vi "Configuration Tool Main.vi"() -> ()   [LabVIEW 2013, in "Configuration Tool.lvlib"]
doc: "This is the main VI for the configuration editor."
uses:
  Configuration Tool.lvlib
  Controls/StateCluster.ctl
  Configuration Framework/Repository/NISE_CEF_Repository.lvclass
  Configuration Framework/Node/NodeRef.ctl
  Configuration Framework/Node/NISE_CEF_Node.lvclass
  Configuration Framework/Node/StandardEvents.ctl
  Configuration Framework/Node/UserEventRef.ctl
  Configuration Framework/Controls/EventCluster.ctl
  Configuration Framework/Node/NodeChangeEvent.ctl
  Configuration Framework/Node/CacheState.ctl
  Configuration Framework/Node/RefreshUIEvent.ctl
  Configuration Framework/Node/StopEvent.ctl
  Configuration Framework/glyph manager/glyph manager.ctl
  <vilib>/picture/picture.llb/imagedata.ctl
  Controls/AddMessage.ctl
  Controls/MoveMessage.ctl
  <vilib>/Utility/error.llb/DialogType.ctl
  Classes/cRIO/cRIO.lvclass
  Classes/cRIO Repo/cRIORepo.lvclass
  <vilib>/Utility/sysdir.llb/System Directory Type.ctl
  <vilib>/NI/AMC/Read Termination Message.vi
  <vilib>/NI/AMC/Create Single Message.vi
  <vilib>/NI/AMC/Update Message Routing Info.vi
  <vilib>/NI/AMC/Send Message.vi
  <vilib>/NI/AMC/Globals.vi
  <vilib>/NI/AMC/AMC.lvlib
  Configuration Framework/NISE_CEF_TreeControl.lvlib
  Configuration Framework/glyph manager/glyph manager.lvlib
panel:
  in  "View":string(tree)
  in  "Exit":bool
  # "Configurator"
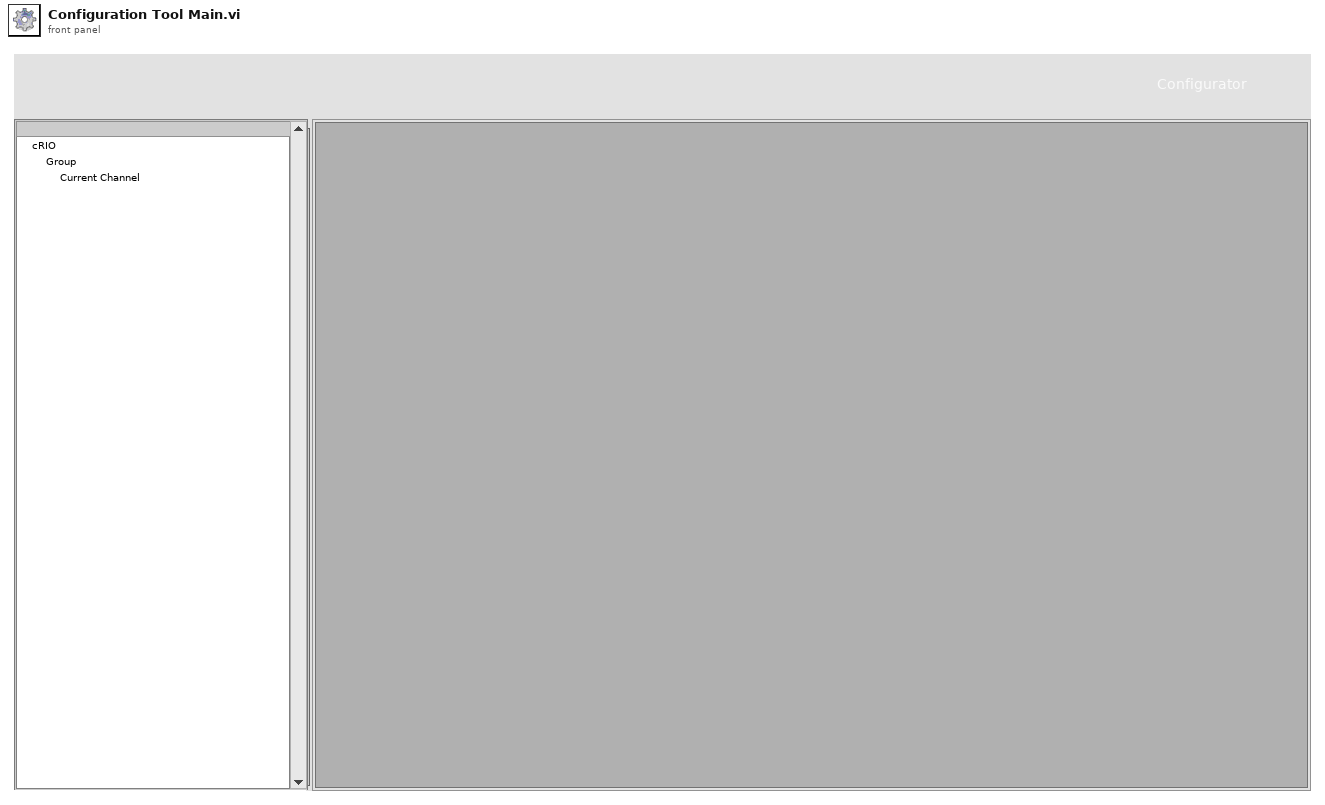
[diagram p1: front panel]
types:
  T1 = typedef "Configuration Tool.lvlib/StateCluster.ctl" = cluster{"repository":refnum<class "NISE_CEF_Repository.lvclass">, "root":T2, "unsaved changes":bool, "current path":path, "standard events":T3, "classes path":path, "glyph manager":T9}
  T2 = typedef "NISE_CEF_Node.lvclass/NodeRef.ctl" = refnum<data-value>
  T3 = typedef "NISE_CEF_Node.lvclass/StandardEvents.ctl" = cluster{"user event":T4, "node change":T5, "cache state":T6, "refresh UI":T7, "stop event":T8}
  T4 = typedef "NISE_CEF_Node.lvclass/UserEventRef.ctl" = refnum<user-event>
  T5 = typedef "NISE_CEF_Node.lvclass/NodeChangeEvent.ctl" = refnum<user-event>
  T6 = typedef "NISE_CEF_Node.lvclass/CacheState.ctl" = refnum<user-event>
  T7 = typedef "NISE_CEF_Node.lvclass/RefreshUIEvent.ctl" = refnum<user-event>
  T8 = typedef "NISE_CEF_Node.lvclass/StopEvent.ctl" = refnum<user-event>
  T9 = typedef "glyph manager.lvlib/glyph manager.ctl" = cluster{"search paths":path[], "glyph map":variant, "base glyphs":T10[], "desired overlays":string[]}
  T10 = typedef "imagedata.ctl" = cluster{"image type":i32, "image depth":i32, "image":u8[], "mask":u8[], "colors":u32[], "Rectangle":cluster{"left":i16, "top":i16, "right":i16, "bottom":i16}}
  T11 = typedef "AMC.lvlib/Message Queue.ctl" = refnum<queue>
  T12 = typedef "Configuration Tool.lvlib/AddMessage.ctl" = cluster{"node type":string, "to add to":string}
  T13 = typedef "Configuration Tool.lvlib/MoveMessage.ctl" = cluster{"node ref":T2, "new parent":T2}
  T14 = typedef "Configuration Tool.lvlib/FilePaths.ctl" = cluster{"glyphs":path, "classes":path}
  T15 = typedef "DialogType.ctl" = u16
  T16 = typedef "System Directory Type.ctl" = i32
  T17 = typedef "NISE_CEF_Node.lvclass/Summary.ctl" = cluster{"ID":string, "parent ID":string, "node type":string, "text":string, "additional text":string, "glyph":string, "depth":i32, "glyph overlay":string}
  T18 = typedef "LVPoint32TypeDef.ctl" = cluster{"Horizontal":i32, "Vertical":i32}
  T19 = cluster{"data name":string, "drag data":variant}[]
  T20 = typedef "NISE_CEF_Node.lvclass/NodeMenuOptions.ctl" = cluster{"removable":bool, "movable":bool, "duplicate":bool}
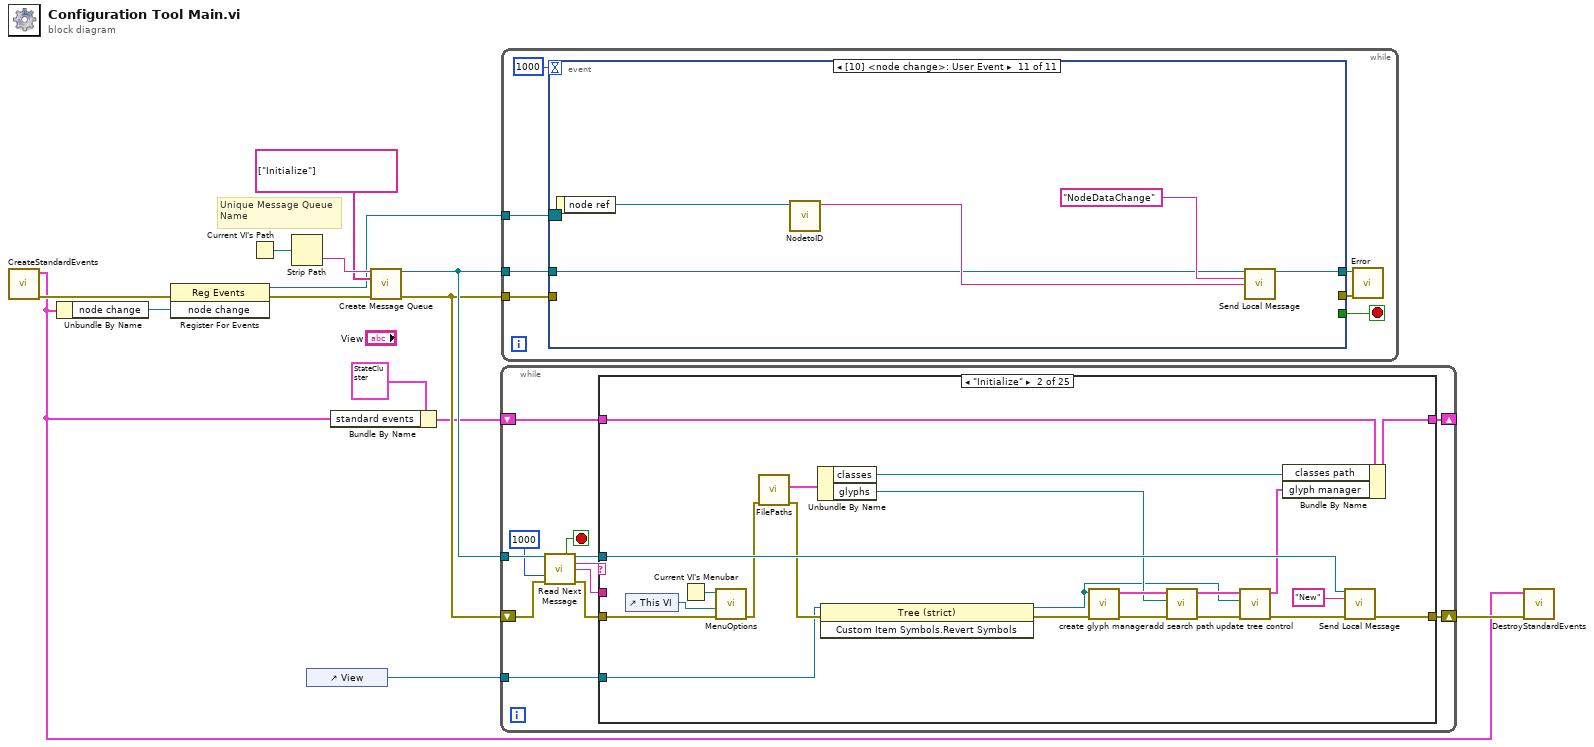
[diagram p0: block diagram]
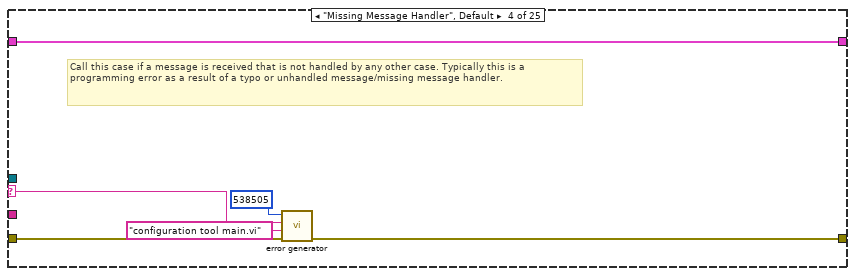
[diagram p4: hidden frame]
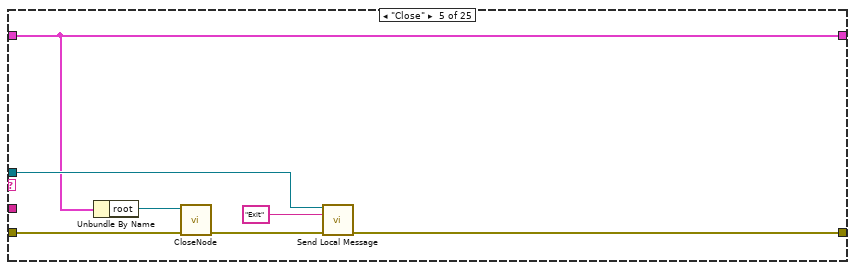
[diagram p5: hidden frame]
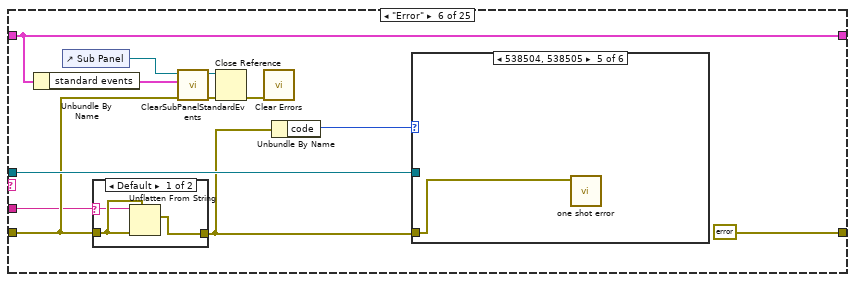
[diagram p6: hidden frame]
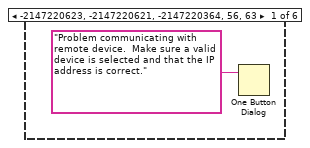
[diagram p8: hidden frame]
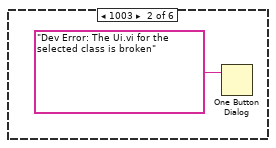
[diagram p9: hidden frame]
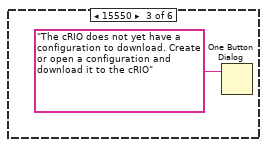
[diagram p10: hidden frame]
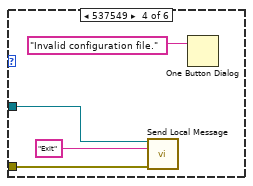
[diagram p11: hidden frame]
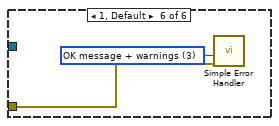
[diagram p12: hidden frame]
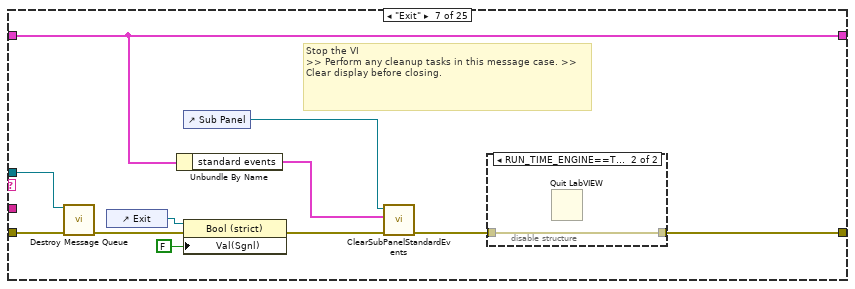
[diagram p13: hidden frame]
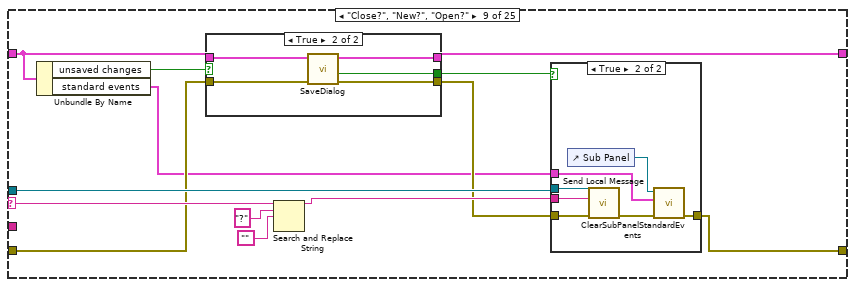
[diagram p16: hidden frame]
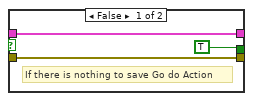
[diagram p17: hidden frame]
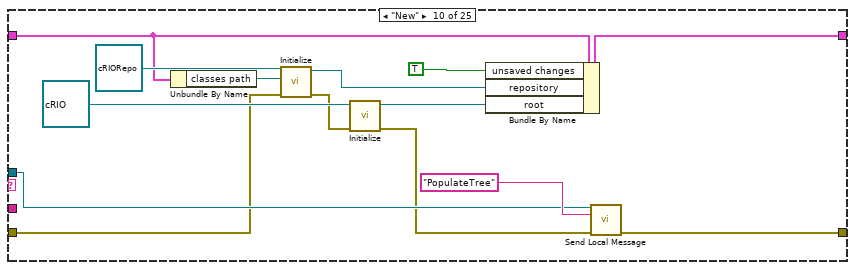
[diagram p19: hidden frame]
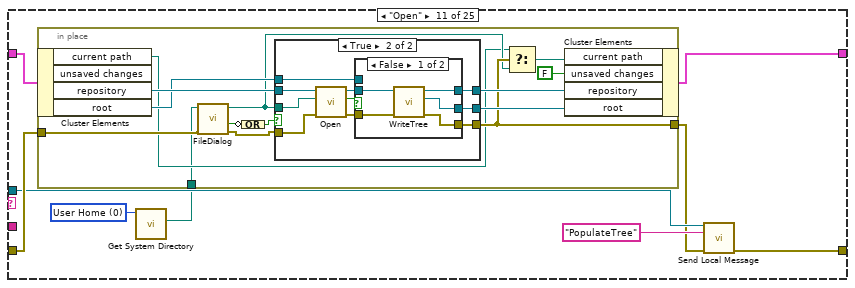
[diagram p20: hidden frame]
diagram:
  # "Unique Message Queue Name"
  n1 = call "CreateStandardEvents.vi"() -> ("error out"=w9:errorcluster, "standard events"=w3:T3)  [unwired: 10 in]
  n2 = Unbundle By Name(w3) -> ("node change"=w8:T5)
  n3 = register-events(error in=w9, w8) -> (reference out=w2:refnum<event-registration>, error out=w7:errorcluster)  [unwired: 1 in]
  n4 = Current VI's Path() -> (path=w13:path)
  n5 = Strip Path(path=w13) -> (name=w14:string)  [unwired: 1 out]
  n6 = control-ref of="View"() -> (w1:refnum<vi>)
  n7 = Bundle By Name(cluster=T1 {"repository"=refnum, "root"=refnum, "unsaved changes"=FALSE, "current path"=path "", "standard events"={"user event"=refnum, "node change"=refnum, "cache state"=refnum, "refresh UI"=refnum, "stop event"=refnum}, "classes path"=path "", "glyph manager"={"search paths"=[], "glyph map"=variant, "base glyphs"=[], "desired overlays"=[]}}, "standard events"=w3) -> (w5:T1)
  n8 = call <vilib>:"Create Message Queue.vi"("message queue name"=w14, "initial message names"=string[] ["Initialize"], "error in"=w7) -> ("message queue out"=w11:T11, "error out"=w10:errorcluster)  [unwired: 11 in]
  n9 = while "Message Processor" {
    shift-right: [w22] -> w4
    shift-left: w10 -> [w21]
    tunnel: w11 -> [w20]
    shift-right: [w18] -> _
    shift-left: w5 -> [w17]
    tunnel: w1 -> [w15]
    stop <- w26 stop-if-true
    n10 = call <vilib>:"Read Next Message.vi"("message queue in"=w20, "timeout (1 ms)"=1000, "error in"=w21) -> ("exit process?"=w26:bool, "message queue out"=w16:T11, "message name"=w25:string, "message value"=w24:string, "error out"=w23:errorcluster)  [unwired: 5 in, 3 out]
    n11 = case shown="\"Initialize\"" w25 {
      selector: w25 -> [_ _ _ w54 _ _ _ _ w115 _ _ _ _ _ _ _ _ w312 _ _ _ _ _ _ _]
      tunnel: w24 -> [_ _ _ _ _ w67 _ _ _ _ _ _ _ w230 _ w273 w290 w310 w349 w373 _ _ w412 w432 w439]
      tunnel: w23 -> [w28 w50 w52 w57 w60 w70 w102 w106 w108 w136 w156 w196 w222 w237 w250 w265 w289 w315 w351 w372 w393 w402 w411 w430 w440]
      tunnel: [w28 w46 w52 w55 w64 errorcluster {"status"=FALSE, "code"=0, "source"=""} ("error out") w94 w106 w119 w148 w152 w200 w224 w234 w250 w267 w293 w318 w354 w369 w387 w398 w408 w425 w438] -> w22
      tunnel: [w27 w42 w51 w58 w62 w74 w93 w105 w110 w146 w157 w203 w223 w231 w249 w259 w286 w319 w353 w374 w383 w401 w406 w433 w435] -> w18
      tunnel: w17 -> [w27 w43 w51 w58 w62 w74 w93 w105 w111 w140 w158 w198 w221 w232 w249 w263 w287 w319 w344 w374 w396 w401 w406 w433 w441]
      tunnel: w16 -> [_ w45 _ _ w63 w77 w101 _ w118 w147 w154 w199 _ w233 _ _ _ w313 _ _ _ _ w407 w424 w437]
      tunnel: w15 -> [_ w29 _ _ _ _ _ _ _ _ _ _ _ _ _ w260 w282 w307 w346 w367 w385 _ _ _ _]
      frame "------------Generic Operations------------" {
        # "Dummy case to add a seperation in the Case Structure menu"
      }
      frame "Initialize" {
        n12 = control-ref of="This VI"() -> (w49:refnum<vi>)
        n13 = Current VI's Menubar() -> (w48:refnum<k9>)
        n14 = call "MenuOptions.vi"("error in"=w50, "VI ref"=w49, "menu ref in"=w48) -> ("error out"=w41:errorcluster)  [unwired: 7 in, 1 out]
        n15 = call "FilePaths.vi"("error in"=w41) -> ("error out"=w32:errorcluster, "paths"=w44:T14)  [unwired: 9 in]
        n16 = Unbundle By Name(w44) -> ("classes"=w40:path, "glyphs"=w34:path)
        n17 = invoke class="Tree (strict)" method="Custom Item Symbols.Revert Symbols"(reference=w29, error in=w32) -> (reference out=w30:refnum<vi>, error out=w31:errorcluster)  [unwired: 1 in, 1 out]
        n18 = call "create glyph manager.vi"("error in"=w31, "tree ref (for default symbols)"=w30) -> ("error out"=w39:errorcluster, "glyph manager"=w38:T9)  [unwired: 8 in]
        n19 = call "add search path.vi"("error in"=w39, "search path"=w34, "glyph manager in"=w38) -> ("error out"=w37:errorcluster, "glyph manager out"=w36:T9)  [unwired: 7 in]
        n20 = call "update tree control.vi"("error in"=w37, "tree reference"=w30, "glyph manager in"=w36) -> ("error out"=w35:errorcluster, "glyph manager out"=w33:T9)  [unwired: 7 in]
        n21 = Bundle By Name(cluster=w43, "classes path"=w40, "glyph manager"=w33) -> (w42:T1)
        n22 = call <vilib>:"Send Local Message.vi"("message queue in"=w45, "message name"="New" ("Message Name"), "error in"=w35) -> ("error out"=w46:errorcluster)  [unwired: 10 in, 2 out]
      }
      frame "", "Idle" {
      }
      frame "Missing Message Handler", Default {
        # "Call this case if a message is received that is not handled by any other case. Typically this is a programming error as a result of a typo or unhandled message/missing message handler."
        n23 = call "error generator.vi"("error in"=w57, "source"="configuration tool main.vi", "append error message"=w54, "error code (0)"=538505) -> ("error out"=w55:errorcluster)  [unwired: 5 in]
      }
      frame "Close" {
        n24 = Unbundle By Name(w62) -> ("root"=w61:T2)
        n25 = call "CloseNode.vi"("error in"=w60, "node ref"=w61) -> ("error out"=w59:errorcluster)  [unwired: 9 in]
        n26 = call <vilib>:"Send Local Message.vi"("message queue in"=w63, "message name"="Exit", "error in"=w59) -> ("error out"=w64:errorcluster)  [unwired: 10 in, 2 out]
      }
      frame "Error" {
        n27 = Unbundle By Name(w74) -> ("standard events"=w66:T3)
        n28 = control-ref of="Sub Panel"() -> (w73:refnum<vi>)
        n29 = case shown="Default" w67 {
          selector: w67 -> [w79 _]
          tunnel: w70 -> [w80 w81]
          tunnel: [w78 w81] -> w69
          frame Default {
            n30 = Unflatten From String(type=w80, binary string=w79, error in (no error)=w80) -> (value=w78:errorcluster)  [unwired: 2 in, 2 out]
          }
          frame "" {
          }
        }
        n31 = call "ClearSubPanelStandardEvents.vi"("error in"=w70, "standard events"=w66, "sub panel ref in"=w73) -> ("error out"=w72:errorcluster, "sub panel ref out"=w71:refnum<vi>)  [unwired: 7 in]
        n32 = Close Reference(reference=w71, error in (no error)=w72) -> (error out=w68:errorcluster)
        n33 = call <vilib>:"Clear Errors.vi"("error in (no error)"=w68) -> ()  [unwired: 6 in, 1 out]
        n34 = Unbundle By Name(w69) -> ("code"=w75:i32)
        n35 = case shown="538504, 538505" w75 {
          tunnel: w77 -> [_ _ _ w87 _ _]
          tunnel: w69 -> [_ _ _ w86 w89 w91]
          frame -2147220623, -2147220621, -2147220364, 56, 63 {
            n36 = One Button Dialog(message="Problem communicating with remote device.  Make sure a valid device is selected and that the IP address is correct.") -> ()  [unwired: 1 in, 1 out]
          }
          frame 1003 {
            n37 = One Button Dialog(message="Dev Error: The Ui.vi for the selected class is broken") -> ()  [unwired: 1 in, 1 out]
          }
          frame 15550 {
            n38 = One Button Dialog(message="The cRIO does not yet have a configuration to download. Create or open a configuration and download it to the cRIO") -> ()  [unwired: 1 in, 1 out]
          }
          frame 537549 {
            n39 = call <vilib>:"Send Local Message.vi"("message queue in"=w87, "message name"="Exit", "error in"=w86) -> ()  [unwired: 10 in, 3 out]
            n40 = One Button Dialog(message="Invalid configuration file.") -> ()  [unwired: 1 in, 1 out]
          }
          frame 538504, 538505 {
            n41 = call "one shot error.vi"("error in"=w89) -> ()  [unwired: 11 in]
          }
          frame 1, Default {
            w90 = T15 3 items=["no dialog", "OK message", "continue or stop message", "OK message + warnings", "continue/stop + warnings"] ("type of dialog (OK msg:1)")
            n42 = call <vilib>:"Simple Error Handler.vi"("type of dialog (OK msg:1)"=w90, "error in (no error)"=w91) -> ()  [unwired: 8 out]
          }
        }
      }
      frame "Exit" {
        # "Stop the VI                                                                             >> Perform any cleanup tasks in this message case. >> Clear display before closing."
        n43 = call <vilib>:"Destroy Message Queue.vi"("message queue in"=w101, "error in"=w102) -> ("error out"=w98:errorcluster)  [unwired: 11 in, 2 out]
        n44 = control-ref of="Exit"() -> (w100:refnum<vi>)
        n45 = Unbundle By Name(w93) -> ("standard events"=w92:T3)
        n46 = control-ref of="Sub Panel"() -> (w97:refnum<vi>)
        n47 = property class="Bool (strict)"(reference=w100, error in=w98, "Val(Sgnl)"=FALSE ("Exit")) -> (error out=w96:errorcluster)  [unwired: 1 out]
        n48 = call "ClearSubPanelStandardEvents.vi"("error in"=w96, "standard events"=w92, "sub panel ref in"=w97) -> ("error out"=w95:errorcluster)  [unwired: 7 in, 1 out]
        n49 = disable-structure shown="RUN_TIME_ENGINE==True" {
          disable-tunnel: [w103 w104] -> w94
          disable-tunnel: w95 -> [w103 w104]
          frame condition #0 (active) {
          }
          frame condition #1 {
            n50 = Quit LabVIEW() -> ()  [unwired: 1 in]
          }
        }
      }
      frame "------------Menu Operations--------------" {
        # "Dummy case to add a seperation in the Case Structure menu"
      }
      frame "Close?", "New?", "Open?" {
        n51 = Unbundle By Name(w111) -> ("unsaved changes"=w113:bool, "standard events"=w107:T3)
        n52 = case shown="True" w113 {
          tunnel: [TRUE ("SaveFlag") w127] -> w112
          tunnel: w111 -> [w121 w126]
          tunnel: [w121 w125] -> w110
          tunnel: w108 -> [w120 w124]
          tunnel: [w120 w123] -> w109
          frame False {
            # "If there is nothing to save Go do Action"
          }
          frame True {
            n53 = call "SaveDialog.vi"("error in"=w124, "state in"=w126) -> ("error out"=w123:errorcluster, "new"=w127:bool, "state out"=w125:T1)  [unwired: 7 in]
          }
        }
        n54 = Search and Replace String(input string=w115, search string="?", replace string="") -> (result string=w114:string)  [unwired: 5 in, 3 out]
        n55 = case shown="True" w112 {
          tunnel: w109 -> [w128 w135]
          tunnel: [w128 w131] -> w119
          tunnel: w118 -> [_ w134]
          tunnel: w114 -> [_ w133]
          tunnel: w107 -> [_ w129]
          frame False {
          }
          frame True {
            n56 = control-ref of="Sub Panel"() -> (w130:refnum<vi>)
            n57 = call <vilib>:"Send Local Message.vi"("message queue in"=w134, "message name"=w133, "error in"=w135) -> ("error out"=w132:errorcluster)  [unwired: 10 in, 2 out]
            n58 = call "ClearSubPanelStandardEvents.vi"("error in"=w132, "standard events"=w129, "sub panel ref in"=w130) -> ("error out"=w131:errorcluster)  [unwired: 7 in, 1 out]
          }
        }
      }
      frame "New" {
        n59 = Unbundle By Name(w140) -> ("classes path"=w139:path)
        n60 = call-dynamic "Initialize.vi"("error in"=w136, "path"=w139, "repository in"=refnum<class "cRIORepo.lvclass"> refnum ("cRIORepo.lvclass")) -> ("error out"=w138:errorcluster, "repository out"=w141:refnum<class "cRIORepo.lvclass">)  [unwired: 7 in]
        n61 = call-dynamic "Initialize.vi"("error in"=w138, "cRIO in"=refnum<class "cRIO.lvclass"> refnum ("cRIO.lvclass")) -> ("error out"=w137:errorcluster, "data value reference"=w143:T2)  [unwired: 7 in, 1 out]
        n62 = Bundle By Name(cluster=w140, "unsaved changes"=TRUE ("SaveFlag"), "repository"=w141, "root"=w143) -> (w146:T1)
        n63 = call <vilib>:"Send Local Message.vi"("message queue in"=w147, "message name"="PopulateTree", "error in"=w137) -> ("error out"=w148:errorcluster)  [unwired: 10 in, 2 out]
      }
      frame "Open" {
        w151 = T16 0 items=["User Home"=0, "User Desktop"=1, "User Documents"=2, "User Application Data"=3, "User Preferences"=4, "User Temporary"=5, "Public Documents"=6, "Public Application Data"=7, "Public Preferences"=8, "Public Cache"=13, "System Core Libraries"=9, "System Installed Libraries"=10, "Application Files"=11, "Boot Volume Root"=12] ("system directory type")
        n64 = call <vilib>:"Get System Directory.vi"("system directory type"=w151) -> ("system directory"=w150:path)  [unwired: 10 in]
        n65 = in-place {
          in-place-border: w156 -> [w164]
          in-place-border: [w163] -> w153
          in-place-border: w150 -> [w159]
          n66 = in-place-cluster #1(w158) -> ("current path"=w161:path, "repository"=w172:refnum<class "NISE_CEF_Repository.lvclass">, "root"=w168:T2)  [unwired: 1 out]
          n67 = call "FileDialog.vi"("error in"=w164, "start path"=w159) -> ("error out"=w165:errorcluster, "cancelled"=w166:bool, "selected path"=w162:path)  [unwired: 7 in]
          n68 = Compound Arithmetic op=OR(invert w166) -> (w167:bool)
          n69 = case shown="True" w167 {
            tunnel: w172 -> [w173 w185]
            tunnel: [w173 w183] -> w170
            tunnel: [w174 w181] -> w163
            tunnel: [w175 w180] -> w169
            tunnel: w162 -> [_ w178]
            tunnel: w165 -> [w174 w177]
            tunnel: w168 -> [w175 w176]
            frame False {
            }
            frame True {
              n70 = call-dynamic "Open.vi"("error in"=w177, "file path"=w178, "repository in"=w185) -> ("error out"=w182:errorcluster, "invalid?"=w179:bool, "repository out"=w184:refnum<class "NISE_CEF_Repository.lvclass">)  [unwired: 6 in]
              n71 = case shown="False" w179 {
                tunnel: w184 -> [w190 w193]
                tunnel: [w189 w193] -> w183
                tunnel: w182 -> [w188 w192]
                tunnel: [w187 w192] -> w181
                tunnel: [w186 w191] -> w180
                tunnel: w176 -> [_ w191]
                frame False {
                  n72 = call-dynamic "WriteTree.vi"("error in"=w188, "repository in"=w190) -> ("error out"=w187:errorcluster, "root"=w186:T2, "repository out"=w189:refnum<class "NISE_CEF_Repository.lvclass">)  [unwired: 7 in]
                }
                frame True {
                }
              }
            }
          }
          n73 = Select(t=w161, s=w163, f=w162) -> (s? t:f=w160:path)
          n74 = in-place-cluster #1("current path"=w160, "unsaved changes"=FALSE ("SaveFlag"), "repository"=w170, "root"=w169) -> (w157:T1)
        }
        n75 = call <vilib>:"Send Local Message.vi"("message queue in"=w154, "message name"="PopulateTree", "error in"=w153) -> ("error out"=w152:errorcluster)  [unwired: 10 in, 2 out]
      }
      frame "Save" {
        n76 = in-place {
          in-place-border: w196 -> [w207]
          in-place-border: [w206] -> w195
          in-place-border: [w204] -> w194
          n77 = in-place-cluster #2(w198) -> ("current path"=w205:path, "root"=w208:T2, "repository"=w210:refnum<class "NISE_CEF_Repository.lvclass">)
          n78 = Empty String/Path?(string/path=w205) -> (empty?=w204:bool)
          n79 = call-dynamic "ReadTree.vi"("error in"=w207, "root"=w208, "repository in"=w210) -> ("error out"=w206:errorcluster, "repository out"=w209:refnum<class "NISE_CEF_Repository.lvclass">)  [unwired: 7 in]
          n80 = in-place-cluster #2("current path"=w205, "root"=w208, "repository"=w209) -> (w197:T1)
        }
        n81 = case shown="True" w194 {
          tunnel: w197 -> [w214 w216]
          tunnel: [w213 w215] -> w203
          tunnel: [w212 w217] -> w201
          tunnel: w195 -> [w211 w218]
          frame False {
            n82 = call "Save.vi"("error in"=w211, "state in"=w214) -> ("error out"=w212:errorcluster, "state out"=w213:T1)  [unwired: 8 in]
          }
          frame True {
            # "Empty path use Dialog"
            n83 = call "SaveAs.vi"("error in"=w218, "state in"=w216) -> ("error out"=w217:errorcluster, "state out"=w215:T1)  [unwired: 7 in, 1 out]
          }
        }
        n84 = call <vilib>:"Send Local Message.vi"("message queue in"=w199, "message name"="PopulateTree", "error in"=w201) -> ("error out"=w200:errorcluster)  [unwired: 10 in, 2 out]
      }
      frame "SaveAs" {
        n85 = in-place {
          in-place-border: w222 -> [w226]
          in-place-border: [w225] -> w220
          n86 = in-place-cluster #3(w221) -> ("root"=w227:T2, "repository"=w229:refnum<class "NISE_CEF_Repository.lvclass">)
          n87 = call-dynamic "ReadTree.vi"("error in"=w226, "root"=w227, "repository in"=w229) -> ("error out"=w225:errorcluster, "repository out"=w228:refnum<class "NISE_CEF_Repository.lvclass">)  [unwired: 7 in]
          n88 = in-place-cluster #3("root"=w227, "repository"=w228) -> (w219:T1)
        }
        n89 = call "SaveAs.vi"("error in"=w220, "state in"=w219) -> ("error out"=w224:errorcluster, "state out"=w223:T1)  [unwired: 7 in, 1 out]
      }
      frame "Custom View" {
        n90 = in-place {
          in-place-border: w237 -> [w248]
          in-place-border: [w247] -> w235
          in-place-border: w230 -> [w238]
          n91 = in-place-cluster #4(w232) -> ("repository"=w242:refnum<class "NISE_CEF_Repository.lvclass">, "root"=w241:T2)
          n92 = call-dynamic "ReadTree.vi"("error in"=w248, "root"=w241, "repository in"=w242) -> ("error out"=w245:errorcluster, "repository out"=w244:refnum<class "NISE_CEF_Repository.lvclass">)  [unwired: 7 in]
          n93 = call-dynamic "CustomView.vi"("error in"=w245, "view name"=w238, "repository in"=w244) -> ("error out"=w246:errorcluster, "repository out"=w243:refnum<class "NISE_CEF_Repository.lvclass">)  [unwired: 7 in]
          n94 = call-dynamic "WriteTree.vi"("error in"=w246, "repository in"=w243) -> ("error out"=w247:errorcluster, "root"=w239:T2, "repository out"=w240:refnum<class "NISE_CEF_Repository.lvclass">)  [unwired: 7 in]
          n95 = in-place-cluster #4("repository"=w240, "root"=w239) -> (w231:T1)
        }
        n96 = call <vilib>:"Send Local Message.vi"("message queue in"=w233, "message name"="PopulateTree", "error in"=w235) -> ("error out"=w234:errorcluster)  [unwired: 10 in, 2 out]
      }
      frame "-------TreeControl Operations-----------" {
        # "Dummy case to add a seperation in the Case Structure menu"
      }
      frame "AddNode" {
        n97 = Unflatten From String(type=T12 {"node type"="", "to add to"=""} ("input cluster"), binary string=w273) -> (value=w271:T12)  [unwired: 3 in, 2 out]
        n98 = Unbundle By Name(w271) -> ("to add to"=w269:string, "node type"=w262:string)
        n99 = in-place {
          in-place-border: w265 -> [w279]
          in-place-border: [w278] -> w264
          in-place-border: w262 -> [w277]
          in-place-border: [w276] -> w261
          n100 = in-place-cluster #5(w263) -> ("repository"=w281:refnum<class "NISE_CEF_Repository.lvclass">)
          n101 = call-dynamic "GetClassPath.vi"("error in"=w279, "class name"=w277, "Repository in"=w281) -> ("error out"=w278:errorcluster, "class path"=w276:path, "Repository out"=w280:refnum<class "NISE_CEF_Repository.lvclass">)  [unwired: 6 in]
          n102 = in-place-cluster #5("repository"=w280) -> (w256:T1)
        }
        n103 = Unbundle By Name(w256) -> ("glyph manager"=w255:T9)
        n104 = call <vilib>:"Get LV Class Default Value.vi"("error in (no error)"=w264, "class path"=w261) -> ("error out"=w274:errorcluster, "object"=w275:refnum<class>)  [unwired: 8 in]
        n105 = To More Specific Class(target class=refnum<class "NISE_CEF_Node.lvclass"> refnum ("Node.lvclass"), reference=w275, error in=w274) -> (specific class reference=w257:refnum<class "NISE_CEF_Node.lvclass">, error out=w258:errorcluster)
        n106 = call-dynamic "AddGlyphtoGManager.vi"("error in"=w258, "glyph manager"=w255, "NISE_CEF_Node in"=w257) -> ("error out"=w253:errorcluster, "glyph manager out"=w254:T9, "NISE_CEF_Node out"=w252:refnum<class "NISE_CEF_Node.lvclass">)  [unwired: 6 in]
        n107 = call "AddNode.vi"("error in"=w253, "node in"=w252, "parent node ID"=w269) -> ("error out"=w268:errorcluster, "summary"=w266:T17[])  [unwired: 7 in]
        n108 = call "PopulateTreeSumaryWithGlyphManager.vi"("error in"=w268, "glyph manager"=w254, "summary"=w266, "tree ref in"=w260) -> ("error out"=w267:errorcluster, "glyph manager out"=w251:T9)  [unwired: 6 in]
        n109 = Bundle By Name(cluster=w256, "glyph manager"=w251) -> (w259:T1)
      }
      frame "Duplicate" {
        n110 = call "IDtoNode.vi"("error in"=w289, "ID"=w290) -> ("error out"=w291:errorcluster, "invalid Id"=w288:bool, "node ref"=w292:T2)  [unwired: 7 in]
        n111 = Unbundle By Name(w287) -> ("glyph manager"=w284:T9)
        n112 = case shown="False" w288 {
          tunnel: [w304 w306] -> w293
          tunnel: w292 -> [w303 _]
          tunnel: w291 -> [w300 w306]
          tunnel: w284 -> [w296 w305]
          tunnel: [w295 w305] -> w283
          tunnel: w282 -> [w294 _]
          frame False {
            n113 = call "DuplicateNode.vi"("same parent?"=TRUE ("s"), "error in"=w300, "node ref in"=w303) -> ("error out"=w301:errorcluster, "new node ref"=w302:T2)  [unwired: 7 in]
            n114 = call "Summary.vi"("error in"=w301, "node self ref"=w302) -> ("error out"=w298:errorcluster, "summary"=w297:T17[])  [unwired: 8 in]
            n115 = call "PopulateTreeSumaryWithGlyphManager.vi"("error in"=w298, "glyph manager"=w296, "summary"=w297, "tree ref in"=w294) -> ("error out"=w304:errorcluster, "glyph manager out"=w295:T9)  [unwired: 6 in]
          }
          frame True {
          }
        }
        n116 = Bundle By Name(cluster=w287, "unsaved changes"=TRUE, "glyph manager"=w283) -> (w286:T1)
      }
      frame "CustomMenuAction" {
        n117 = Match Pattern(string=w310, regular expression=":") -> (before substring=w309:string, after substring=w308:string)  [unwired: 1 in, 2 out]
        n118 = call "IDtoNode.vi"("error in"=w315, "ID"=w308) -> ("error out"=w316:errorcluster, "invalid Id"=w314:bool, "node ref"=w317:T2)  [unwired: 7 in]
        n119 = case shown="False" w314 {
          tunnel: [w322 w342] -> w318
          tunnel: w317 -> [w327 _]
          tunnel: w316 -> [w325 w342]
          tunnel: w313 -> [w326 _]
          tunnel: w312 -> [_ _]
          tunnel: w309 -> [w323 _]
          tunnel: w307 -> [w320 _]
          frame False {
            n120 = in-place {
              in-place-border: w326 -> [w340]
              in-place-border: w325 -> [w338]
              in-place-border: [w337] -> w321
              in-place-border: [w336] -> w324
              in-place-border: w323 -> [w335]
              in-place-border: w320 -> [w334]
              n121 = in-place-dvr #6(w327) -> (w341:refnum<class "NISE_CEF_Node.lvclass">)  [unwired: 1 out]
              n122 = call-dynamic "MenuHandler.vi"("tree control"=w334, "main message queue"=w340, "error in"=w338, "menu string"=w335, "NISE_CEF_Node in"=w341) -> ("error out"=w337:errorcluster, "Unhandled"=w336:bool, "NISE_CEF_Node out"=w339:refnum<class "NISE_CEF_Node.lvclass">)  [unwired: 4 in]
              n123 = in-place-dvr #6(w339) -> ()  [unwired: 2 out]
            }
            n124 = case shown="True" w324 {
              tunnel: w323 -> [_ w329]
              tunnel: [w328 w330] -> w322
              tunnel: w321 -> [w328 w331]
              frame False {
              }
              frame True {
                n125 = call "error generator.vi"("error in"=w331, "source"="configuration tool main.vi", "append error message"=w329, "error code (0)"=538506) -> ("error out"=w330:errorcluster)  [unwired: 5 in]
              }
            }
          }
          frame True {
          }
        }
      }
      frame "RefreshNode" {
        # "Refreshes the node in the Tree, Sets the save flag to true. This case can be called from the UIs of the nodes"
        n126 = Unbundle By Name(w344) -> ("glyph manager"=w343:T9)
        n127 = call "IDtoNode.vi"("error in"=w351, "ID"=w349) -> ("error out"=w350:errorcluster, "invalid Id"=w347:bool, "node ref"=w348:T2)  [unwired: 7 in]
        n128 = case shown="True" w347 {
          tunnel: [w363 w366] -> w354
          tunnel: w350 -> [w359 w366]
          tunnel: w348 -> [w358 _]
          tunnel: w346 -> [w357 _]
          tunnel: [w356 w365] -> w345
          tunnel: w343 -> [w355 w365]
          frame False {
            n129 = call "Summary.vi"("error in"=w359, "node self ref"=w358) -> ("error out"=w361:errorcluster, "summary"=w360:T17[])  [unwired: 8 in]
            n130 = call "RefreshSubTreeWithGlyphManager.vi"("error in"=w361, "glyph manager"=w355, "node information"=w360, "tree ref in"=w357) -> ("error out"=w364:errorcluster, "glyph manager out"=w356:T9, "tree ref out"=w362:refnum<vi>)  [unwired: 5 in]
            n131 = Close Reference(reference=w362, error in (no error)=w364) -> (error out=w363:errorcluster)
          }
          frame True {
          }
        }
        n132 = Bundle By Name(cluster=w344, "unsaved changes"=TRUE ("SaveFlag"), "glyph manager"=w345) -> (w353:T1)
      }
      frame "RemoveNode" {
        n133 = call "IDtoNode.vi"("error in"=w372, "ID"=w373) -> ("error out"=w371:errorcluster, "invalid Id"=w368:bool, "node ref"=w370:T2)  [unwired: 7 in]
        n134 = case shown="False" w368 {
          tunnel: w371 -> [w380 w381]
          tunnel: w370 -> [w379 _]
          tunnel: [w376 w381] -> w369
          tunnel: w367 -> [w375 _]
          frame False {
            n135 = call "RemoveNode.vi"("error in"=w380, "node"=w379) -> ("error out"=w377:errorcluster, "node ID"=w378:string)  [unwired: 8 in]
            n136 = call "ClearTreeNode.vi"("error in"=w377, "tag"=w378, "tree reference"=w375) -> ("error out"=w376:errorcluster)  [unwired: 8 in]
          }
          frame True {
          }
        }
      }
      frame "PopulateTree" {
        n137 = Unbundle By Name(w396) -> ("standard events"=w386:T3, "glyph manager"=w384:T9, "root"=w391:T2)
        n138 = call "Summary.vi"("error in"=w393, "depth"=0 ("Depth"), "node self ref"=w391) -> ("error out"=w392:errorcluster, "summary"=w395:T17[])  [unwired: 7 in]
        n139 = control-ref of="This VI"() -> (w394:refnum<vi>)
        n140 = call "RefreshEntireTreeWithGlyphManager.vi"("calling VI in"=w394, "error in"=w392, "glyph manager"=w384, "array"=w395, "tree ref in"=w385) -> ("error out"=w388:errorcluster, "glyph manager out"=w382:T9)  [unwired: 5 in]
        n141 = control-ref of="Sub Panel"() -> (w389:refnum<vi>)
        n142 = Bundle By Name(cluster=w396, "glyph manager"=w382) -> (w383:T1)
        n143 = call "ClearSubPanelStandardEvents.vi"("error in"=w388, "standard events"=w386, "sub panel ref in"=w389) -> ("error out"=w387:errorcluster)  [unwired: 7 in, 1 out]
      }
      frame "CleansubPanel" {
        n144 = Unbundle By Name(w401) -> ("standard events"=w397:T3)
        n145 = control-ref of="Sub Panel"() -> (w403:refnum<vi>)
        n146 = call "ClearSubPanelStandardEvents.vi"("error in"=w402, "standard events"=w397, "sub panel ref in"=w403) -> ("error out"=w400:errorcluster, "sub panel ref out"=w399:refnum<vi>)  [unwired: 7 in]
        n147 = Close Reference(reference=w399, error in (no error)=w400) -> (error out=w398:errorcluster)
      }
      frame "ActivateNode" {
        n148 = Unbundle By Name(w406) -> ("standard events"=w405:T3)
        n149 = call "IDtoNode.vi"("error in"=w411, "ID"=w412) -> ("error out"=w404:errorcluster, "invalid Id"=w410:bool, "node ref"=w409:T2)  [unwired: 7 in]
        n150 = case shown="False" w410 {
          tunnel: w409 -> [w419 _]
          tunnel: [w420 w421] -> w408
          tunnel: w404 -> [w417 w421]
          tunnel: w407 -> [w415 _]
          tunnel: w405 -> [w413 _]
          frame False {
            n151 = control-ref of="Sub Panel"() -> (w416:refnum<vi>)
            n152 = call "ClearSubPanelStandardEvents.vi"("error in"=w417, "standard events"=w413, "sub panel ref in"=w416) -> ("error out"=w418:errorcluster, "sub panel ref out"=w414:refnum<vi>)  [unwired: 7 in]
            n153 = call "LoadNodeUIStandardEvents.vi"("user event out"=w413, "error in"=w418, "sub panel ref in"=w414, "main queue"=w415, "node"=w419) -> ("error out"=w420:errorcluster)  [unwired: 6 in]
          }
          frame True {
          }
        }
      }
      frame "Move" {
        n154 = Unflatten From String(type=T13 {"node ref"=refnum, "new parent"=refnum} ("Cluster"), binary string=w432, error in (no error)=w430) -> (value=w429:T13, error out=w428:errorcluster)  [unwired: 2 in, 1 out]
        n155 = Unbundle By Name(w429) -> ("node ref"=w423:T2, "new parent"=w422:T2)
        n156 = call "MoveNode.vi"("error in"=w428, "new parent"=w422, "node"=w423) -> ("error out"=w426:errorcluster)  [unwired: 8 in]
        n157 = call <vilib>:"Send Local Message.vi"("message queue in"=w424, "message name"="PopulateTree", "error in"=w426) -> ("error out"=w425:errorcluster)  [unwired: 10 in, 2 out]
      }
      frame "NodeDataChange" {
        n158 = call <vilib>:"Send Local Message.vi"("message queue in"=w437, "message name"="RefreshNode", "message value"=w439, "error in"=w440) -> ("error out"=w438:errorcluster)  [unwired: 9 in, 2 out]
        n159 = Bundle By Name(cluster=w441, "unsaved changes"=TRUE) -> (w435:T1)
      }
    }
  }
  n160 = while "User Interface Event Handler" {
    tunnel: w11 -> [w447]
    tunnel: w10 -> [w443]
    tunnel: w2 -> [w442]
    stop <- w446 stop-if-true
    n161 = event shown="[10] <node change>: User Event" {
      selector: w442 -> [_ _ _ _ _ _ _ _ _ _ _]
      dyn-events: _ -> [_ _ _ _ _ _ _ _ _ _ _]
      timeout: 1000 -> [_ _ _ _ _ _ _ _ _ _ _]
      tunnel: w447 -> [w450 w458 w482 w534 w562 w569 w598 w602 w612 w618 w664]
      tunnel: [_ _ _ _ TRUE _ _ _ _ _ _] -> w446
      tunnel: [w450 w458 w479 w532 w558 w569 w595 w602 w610 w617 w665] -> w445
      tunnel: [w449 w454 w478 w531 w559 w565 w594 w599 w608 w615 _] -> w444
      tunnel: w443 -> [w449 w457 w477 w533 w560 w568 w593 w601 w609 w616 _]
      event Timeout {
        # "Timeout code can be added here for autosave or Lock Screen"
        n162 = event-data() -> ()  [unwired: 1 in, 1 out]
      }
      event "View": Shortcut Menu Activation? {
        n163 = event-data() -> ("CtlRef"=w464:refnum<vi>, "Coords"=w463:T18, "MenuRef"=w460:refnum<k9>)  [unwired: 1 in]
        n164 = invoke class="Tree (strict)" method="Point To Row Column"(reference=w464, error in=w457, "Point"=w463) -> (error out=w456:errorcluster, "Tag"=w462:string)  [unwired: 5 in, 6 out]
        n165 = call "IDtoNode.vi"("error in"=w456, "ID"=w462) -> ("error out"=w452:errorcluster, "invalid Id"=w459:bool, "node ref"=w461:T2)  [unwired: 7 in]
        n166 = case shown="False" w459 {
          tunnel: w461 -> [w469 _]
          tunnel: w460 -> [w468 _]
          tunnel: [w467 _] -> w455
          tunnel: [w466 _] -> w453
          tunnel: w452 -> [w465 w475]
          tunnel: [w465 w475] -> w451
          frame False {
            n167 = in-place {
              in-place-border: w468 -> [w472]
              in-place-border: [w470] -> w467
              n168 = in-place-dvr #7(w469) -> (w474:refnum<class "NISE_CEF_Node.lvclass">, w471:errorcluster)
              n169 = call-dynamic "ShortcutMenu.vi"("error in"=w471, "menu ref in"=w472, "node in"=w474) -> ("error out"=w470:errorcluster, "node out"=w473:refnum<class "NISE_CEF_Node.lvclass">)  [unwired: 6 in, 1 out]
              n170 = in-place-dvr #7(w473) -> (w466:errorcluster)  [unwired: 1 out]
            }
          }
          frame True {
          }
        }
        n171 = Merge Errors(w453, w455, w451) -> (w454:errorcluster)
        n172 = event-data() -> ()  [unwired: 2 in, 1 out]
      }
      event "View": Shortcut Menu Selection (User) {
        n173 = event-data() -> ("ItemPath"=w481:string, "CtlRef"=w485:refnum<vi>, "Coords"=w486:T18)  [unwired: 1 in]
        n174 = invoke class="Tree (strict)" method="Point To Row Column"(reference=w485, error in=w477, "Point"=w486) -> (error out=w476:errorcluster, "Tag"=w480:string)  [unwired: 5 in, 6 out]
        n175 = Match Pattern(string=w481, regular expression=":") -> (before substring=w484:string, after substring=w483:string)  [unwired: 1 in, 2 out]
        n176 = case shown="Default" w484 {
          selector: w484 -> [w488 _ _ _]
          tunnel: w483 -> [_ _ _ w513]
          tunnel: w482 -> [w495 w502 w508 w515]
          tunnel: w480 -> [w490 w500 w506 w514]
          tunnel: [w492 w499 w505 w511] -> w479
          tunnel: [w493 w498 w503 w509] -> w478
          tunnel: w476 -> [w494 w497 w504 w510]
          frame Default {
            n177 = Concatenate Strings(w488, ":" ("string"), w490) -> (w491:string)
            n178 = call <vilib>:"Send Local Message.vi"("message queue in"=w495, "message name"="CustomMenuAction" ("Message Name"), "message value"=w491, "error in"=w494) -> ("message queue out"=w492:T11, "error out"=w493:errorcluster)  [unwired: 9 in, 1 out]
          }
          frame "Remove" {
            n179 = call <vilib>:"Send Local Message.vi"("message queue in"=w502, "message name"="RemoveNode" ("Message Name"), "message value"=w500, "error in"=w497) -> ("message queue out"=w499:T11, "error out"=w498:errorcluster)  [unwired: 9 in, 1 out]
          }
          frame "Duplicate" {
            n180 = call <vilib>:"Send Local Message.vi"("message queue in"=w508, "message name"="Duplicate" ("Message Name"), "message value"=w506, "error in"=w504) -> ("message queue out"=w505:T11, "error out"=w503:errorcluster)  [unwired: 9 in, 1 out]
          }
          frame "Add" {
            n181 = Bundle By Name(cluster=T12 {"node type"="", "to add to"=""} ("input cluster"), "node type"=w513, "to add to"=w514) -> (w516:T12)
            n182 = Flatten To String(anything=w516) -> (data string=w517:string)  [unwired: 3 in, 2 out]
            n183 = call <vilib>:"Send Local Message.vi"("message queue in"=w515, "message name"="AddNode" ("Message Name"), "message value"=w517, "error in"=w510) -> ("message queue out"=w511:T11, "error out"=w509:errorcluster)  [unwired: 9 in, 1 out]
          }
        }
      }
      event "View": Drop {
        n184 = event-data() -> ("CtlRef"=w537:refnum<vi>, "Coords"=w536:T18)  [unwired: 1 in]
        n185 = invoke class="Tree (strict)" method="Point To Row Column"(reference=w537, error in=w533, "Point"=w536) -> (reference out=w535:refnum<vi>, error out=w530:errorcluster, "Tag"=w527:string)  [unwired: 5 in, 5 out]
        n186 = call "ValidDragDrop.vi"("error in"=w530, "drag over"=w527, "tree ref in"=w535) -> ("error out"=w522:errorcluster, "accepted"=w525:bool, "drag"=w529:string, "tree ref out"=w539:refnum<vi>)  [unwired: 5 in]
        n187 = call "IDtoNode.vi"("error in"=w522, "ID"=w527) -> ("error out"=w523:errorcluster, "invalid Id"=w520:bool, "node ref"=w526:T2)  [unwired: 7 in]
        n188 = call "IDtoNode.vi"("error in"=w523, "ID"=w529) -> ("error out"=w521:errorcluster, "invalid Id"=w519:bool, "node ref"=w528:T2)  [unwired: 7 in]
        n189 = Compound Arithmetic op=AND(w525, invert w520, invert w519) -> (w524:bool)
        n190 = case shown="True" w524 {
          tunnel: w529 -> [_ w555]
          tunnel: w539 -> [_ w557]
          tunnel: [_ TRUE] -> w538
          tunnel: w527 -> [_ w553]
          tunnel: w534 -> [w541 w552]
          tunnel: [w541 w548] -> w532
          tunnel: [w540 w547] -> w531
          tunnel: w528 -> [_ w543]
          tunnel: w526 -> [_ w542]
          tunnel: w521 -> [w540 w544]
          frame False {
          }
          frame True {
            n191 = invoke class="Tree (strict)" method="Edit Tree Items.Move Item"(reference=w557, error in=w544, "tag"=w555, "New Parent"=w553) -> (error out=w545:errorcluster)  [unwired: 3 in, 6 out]
            n192 = Bundle By Name(cluster=T13 {"node ref"=refnum, "new parent"=refnum} ("Cluster"), "new parent"=w542, "node ref"=w543) -> (w551:T13)
            n193 = Flatten To String(anything=w551, error in (no error)=w545) -> (data string=w550:string, error out=w546:errorcluster)  [unwired: 2 in, 1 out]
            n194 = call <vilib>:"Send Local Message.vi"("message queue in"=w552, "message name"="Move", "message value"=w550, "error in"=w546) -> ("message queue out"=w548:T11, "error out"=w547:errorcluster)  [unwired: 9 in, 1 out]
          }
        }
        n195 = event-data("Accepted?"=w538) -> ()  [unwired: 1 in, 1 out]
      }
      event "Exit": Value Change {
        # "Exit the application                                           >> Stop this message generator loop    Cleaning errors if the other loop stop this one"
        n196 = event-data() -> ()  [unwired: 1 in, 1 out]
        n197 = call <vilib>:"Send Local Message.vi"("message queue in"=w562, "message name"="Close", "error in"=w560) -> ("message queue out"=w558:T11, "error out"=w563:errorcluster)  [unwired: 10 in, 1 out]
        n198 = call <vilib>:"Clear Errors.vi"("error in (no error)"=w563) -> ("error out"=w559:errorcluster)  [unwired: 6 in]
      }
      event "View": Drag Starting? {
        n199 = event-data() -> ("Data"=w575:T19, "CtlRef"=w577:refnum<vi>, "Coords"=w576:T18)  [unwired: 1 in]
        n200 = invoke class="Tree (strict)" method="Point To Row Column"(reference=w577, error in=w568, "Point"=w576) -> (error out=w567:errorcluster, "Tag"=w574:string)  [unwired: 5 in, 6 out]
        n201 = call "IDtoNode.vi"("error in"=w567, "ID"=w574) -> ("error out"=w566:errorcluster, "invalid Id"=w573:bool, "node ref"=w572:T2)  [unwired: 7 in]
        n202 = case shown="False" w573 {
          tunnel: w572 -> [w585 _]
          tunnel: [w582 TRUE ("Removable")] -> w570
          tunnel: w566 -> [w581 w591]
          tunnel: [w578 w591] -> w565
          frame False {
            n203 = in-place {
              in-place-border: [w588] -> w584
              in-place-border: w581 -> [w587]
              in-place-border: [w586] -> w580
              n204 = in-place-dvr #8(w585) -> (w590:refnum<class "NISE_CEF_Node.lvclass">)  [unwired: 1 out]
              n205 = call-dynamic "EditOptions.vi"("error in"=w587, "node in"=w590) -> ("error out"=w586:errorcluster, "edit options"=w588:T20, "node out"=w589:refnum<class "NISE_CEF_Node.lvclass">)  [unwired: 6 in, 1 out]
              n206 = in-place-dvr #8(w589) -> (w579:errorcluster)  [unwired: 1 out]
            }
            n207 = Unbundle By Name(w584) -> ("movable"=w583:bool)
            n208 = Merge Errors(w579, w580) -> (w578:errorcluster)
            n209 = Not(x=w583) -> (.not. x?=w582:bool)
          }
          frame True {
          }
        }
        n210 = event-data("Data"=w575, "Drag Mode"=enum32{"copy or move", "copy only", "move only"}."move only", "Discard?"=w570) -> ()  [unwired: 1 in, 1 out]
      }
      event "View": Value Change {
        n211 = event-data() -> ("NewVal"=w596:string)  [unwired: 1 in]
        n212 = call <vilib>:"Send Local Message.vi"("message queue in"=w598, "message name"="ActivateNode" ("Message Name"), "message value"=w596, "error in"=w593) -> ("message queue out"=w595:T11, "error out"=w594:errorcluster)  [unwired: 9 in, 1 out]
      }
      event "View": event type 3.0.xa000003a {
        n213 = event-data() -> ("CtlRef"=w607:refnum<vi>, "Coords"=w604:T18)  [unwired: 1 in]
        n214 = invoke class="Tree (strict)" method="Point To Row Column"(reference=w607, error in=w601, "Point"=w604) -> (reference out=w606:refnum<vi>, error out=w600:errorcluster, "Tag"=w605:string)  [unwired: 5 in, 5 out]
        n215 = call "ValidDragDrop.vi"("error in"=w600, "drag over"=w605, "tree ref in"=w606) -> ("error out"=w599:errorcluster, "accepted"=w603:bool)  [unwired: 5 in, 2 out]
        n216 = event-data("Accepted?"=w603) -> ()  [unwired: 1 in, 1 out]
      }
      event Panel Close? {
        # "Intercepts the upper right close panel operation to allow a smooth shutdown as opposed to immediately killing the app."
        n217 = event-data() -> ()  [unwired: 1 in, 1 out]
        n218 = call <vilib>:"Send Local Message.vi"("message queue in"=w612, "message name"="Close?", "error in"=w609) -> ("message queue out"=w610:T11, "error out"=w608:errorcluster)  [unwired: 10 in, 1 out]
        n219 = event-data("Discard?"=TRUE) -> ()  [unwired: 1 in, 1 out]
      }
      event Menu Selection (User) {
        # "#USERCFG It is needed to add a Case for Every item on the menu"
        n220 = event-data() -> ("ItemTag"=w614:string, "ItemPath"=w619:string)  [unwired: 1 in]
        n221 = case shown="Default" w619 {
          selector: w619 -> [w623 _ _ _ _ _ _]
          tunnel: w618 -> [w628 w633 w638 w643 w648 w653 w662]
          tunnel: [w628 w629 w634 w639 w644 w649 w659] -> w617
          tunnel: w616 -> [w625 w631 w636 w641 w646 w651 w658]
          tunnel: [w624 w630 w635 w640 w645 w650 w656] -> w615
          tunnel: w614 -> [w622 _ _ _ _ _ _]
          frame Default {
            n222 = Concatenate Strings(w622, "::" ("string"), w623) -> (w621:string)
            n223 = call "error generator.vi"("error in"=w625, "source"="configuration tool main.vi", "append error message"=w621, "error code (0)"=538506) -> ("error out"=w624:errorcluster)  [unwired: 5 in]
          }
          frame "_File:_New" {
            n224 = call <vilib>:"Send Local Message.vi"("message queue in"=w633, "message name"="New?" ("Message Name"), "error in"=w631) -> ("message queue out"=w629:T11, "error out"=w630:errorcluster)  [unwired: 10 in, 1 out]
          }
          frame "_File:_Open" {
            n225 = call <vilib>:"Send Local Message.vi"("message queue in"=w638, "message name"="Open?" ("Message Name"), "error in"=w636) -> ("message queue out"=w634:T11, "error out"=w635:errorcluster)  [unwired: 10 in, 1 out]
          }
          frame "_File:_Save" {
            n226 = call <vilib>:"Send Local Message.vi"("message queue in"=w643, "message name"="Save" ("Message Name"), "error in"=w641) -> ("message queue out"=w639:T11, "error out"=w640:errorcluster)  [unwired: 10 in, 1 out]
          }
          frame "_File:Save As..." {
            n227 = call <vilib>:"Send Local Message.vi"("message queue in"=w648, "message name"="SaveAs" ("Message Name"), "error in"=w646) -> ("message queue out"=w644:T11, "error out"=w645:errorcluster)  [unwired: 10 in, 1 out]
          }
          frame "_File:_Exit" {
            n228 = call <vilib>:"Send Local Message.vi"("message queue in"=w653, "message name"="Close?" ("Message Name"), "error in"=w651) -> ("message queue out"=w649:T11, "error out"=w650:errorcluster)  [unwired: 10 in, 1 out]
          }
          frame "_Tools:Multiple Parameter Editor" {
            n229 = call <vilib>:"Send Local Message.vi"("message queue in"=w662, "message name"="CleansubPanel", "error in"=w658) -> ("message queue out"=w661:T11, "error out"=w657:errorcluster)  [unwired: 10 in, 1 out]
            n230 = call <vilib>:"Send Local Message.vi"("message queue in"=w661, "message name"="Custom View" ("Message Name"), "message value"="Multiple Variable Editor" ("Message Name"), "error in"=w657) -> ("message queue out"=w659:T11, "error out"=w656:errorcluster)  [unwired: 9 in, 1 out]
          }
        }
      }
      event User Event {
        n231 = event-data() -> ("node ref"=w663:T2)  [unwired: 1 in]
        n232 = call "NodetoID.vi"("node ref"=w663) -> ("ID"=w666:string)  [unwired: 9 in, 1 out]
        n233 = call <vilib>:"Send Local Message.vi"("message queue in"=w664, "message name"="NodeDataChange", "message value"=w666) -> ("message queue out"=w665:T11)  [unwired: 10 in, 2 out]
      }
    }
    n234 = call "Error.vi"("error in (no error)"=w444, "message queue in"=w445) -> ()  [unwired: 9 in, 1 out]
  }
  n235 = call "DestroyStandardEvents.vi"("error in"=w4, "standard events"=w3) -> ()  [unwired: 9 in, 1 out]
